vi "InjectObjectReference.vi"(6 "Dynamic Dispatch":bool, 8 "error in (no error)":errorcluster, 11 "CreateClass In":refnum<class "CreateClass.lvclass">) -> (0 "error out":errorcluster, 3 "CreateClass Out":refnum<class "CreateClass.lvclass">)   [LabVIEW 2020, in "Mermaid.lvlib" / "CreateClass.lvclass"]
uses:
  CreateClass.lvclass
  CreateClass.lvclass/CreateClass.ctl
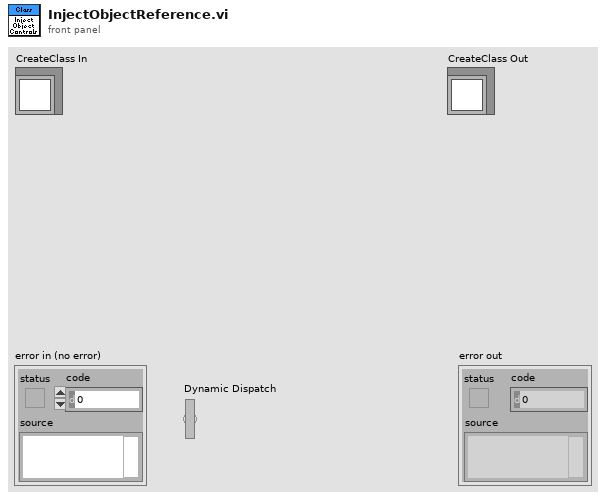
[diagram p1: front panel]
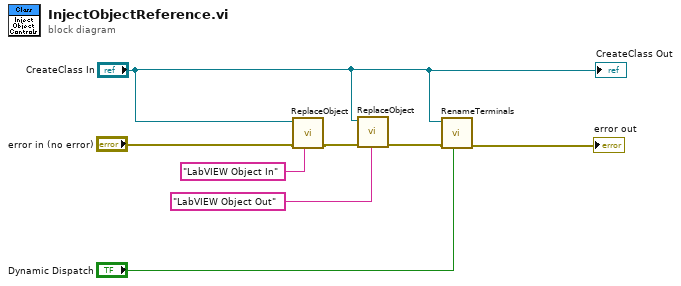
[diagram p0: block diagram]
diagram:
  n1 = call "ReplaceObject.vi"("name/order"="LabVIEW Object In", "error in (no error)"="error in (no error)", "CreateClass In"="CreateClass In") -> ("error out"=w5:errorcluster)  [unwired: 8 in]
  n2 = call "ReplaceObject.vi"("name/order"="LabVIEW Object Out", "error in (no error)"=w5, "CreateClass In"="CreateClass In") -> ("error out"=w4:errorcluster)  [unwired: 8 in]
  n3 = call "RenameTerminals.vi"("Dynamic Dispatch"="Dynamic Dispatch", "error in (no error)"=w4, "CreateClass In"="CreateClass In") -> ("error out"=→"error out":errorcluster)  [unwired: 8 in]
  "CreateClass Out" <- "CreateClass In"
